vi "purge_v01.vi"(2 "Debug Mode":bool, 3 "Elapsed Time(s)":dbl, 4 "State":enum16{"Edit", "Start", "Run", "End", "Idle"}(ring), 5 "Argument List In":string[](array[string])) -> (0 "Status Out":string, 1 "Argument List Out":string[](array[string]))   [LabVIEW 2011]
panel:
  out "first":bool=TRUE
  out "total time":dbl
  out "is OK?":bool
  out "AsH3?":bool
  out "PH3?":bool
  out "In?":bool
  out "Ga?":bool
  out "Al?":bool
  in  "AsH3 Flow":dbl caption="AsH3 Flow (0-10 sccm)" format="%.2f"
  in  "P Flow":dbl caption="P Flow (0-100 sccm)" format="%.2f"
  in  "In Flow":dbl caption="In Flow (0-100 sscm)" format="%.2f"
  in  "Ga Flow":dbl caption="Ga Flow (0-10 sscm)" format="%.2f"
  in  "Al Flow":dbl caption="Al Flow (0-100 sscm)" format="%.2f"
  in  "Cancel":bool
  in  "OK":bool
  out "tTotal(s) 2":dbl
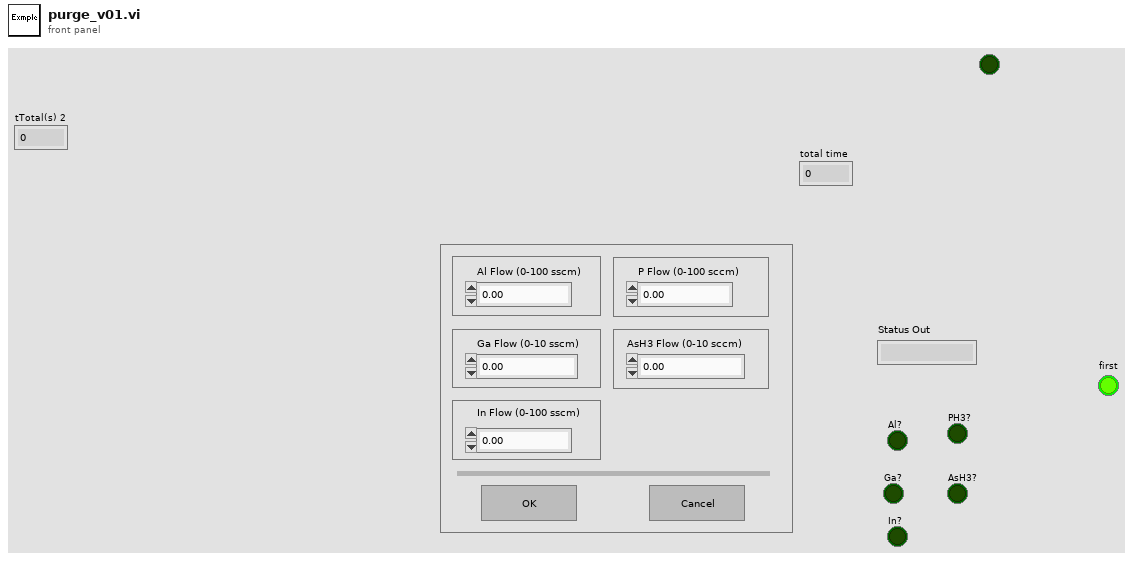
[diagram p1: front panel]
types:
  T1 = enum16{"Discrete", "Continuous", "Instantaneous", "Finite"}
  T2 = enum32{"Invalid", "Default", "Floating", "Floating/Auto-Hide", "Modal"}
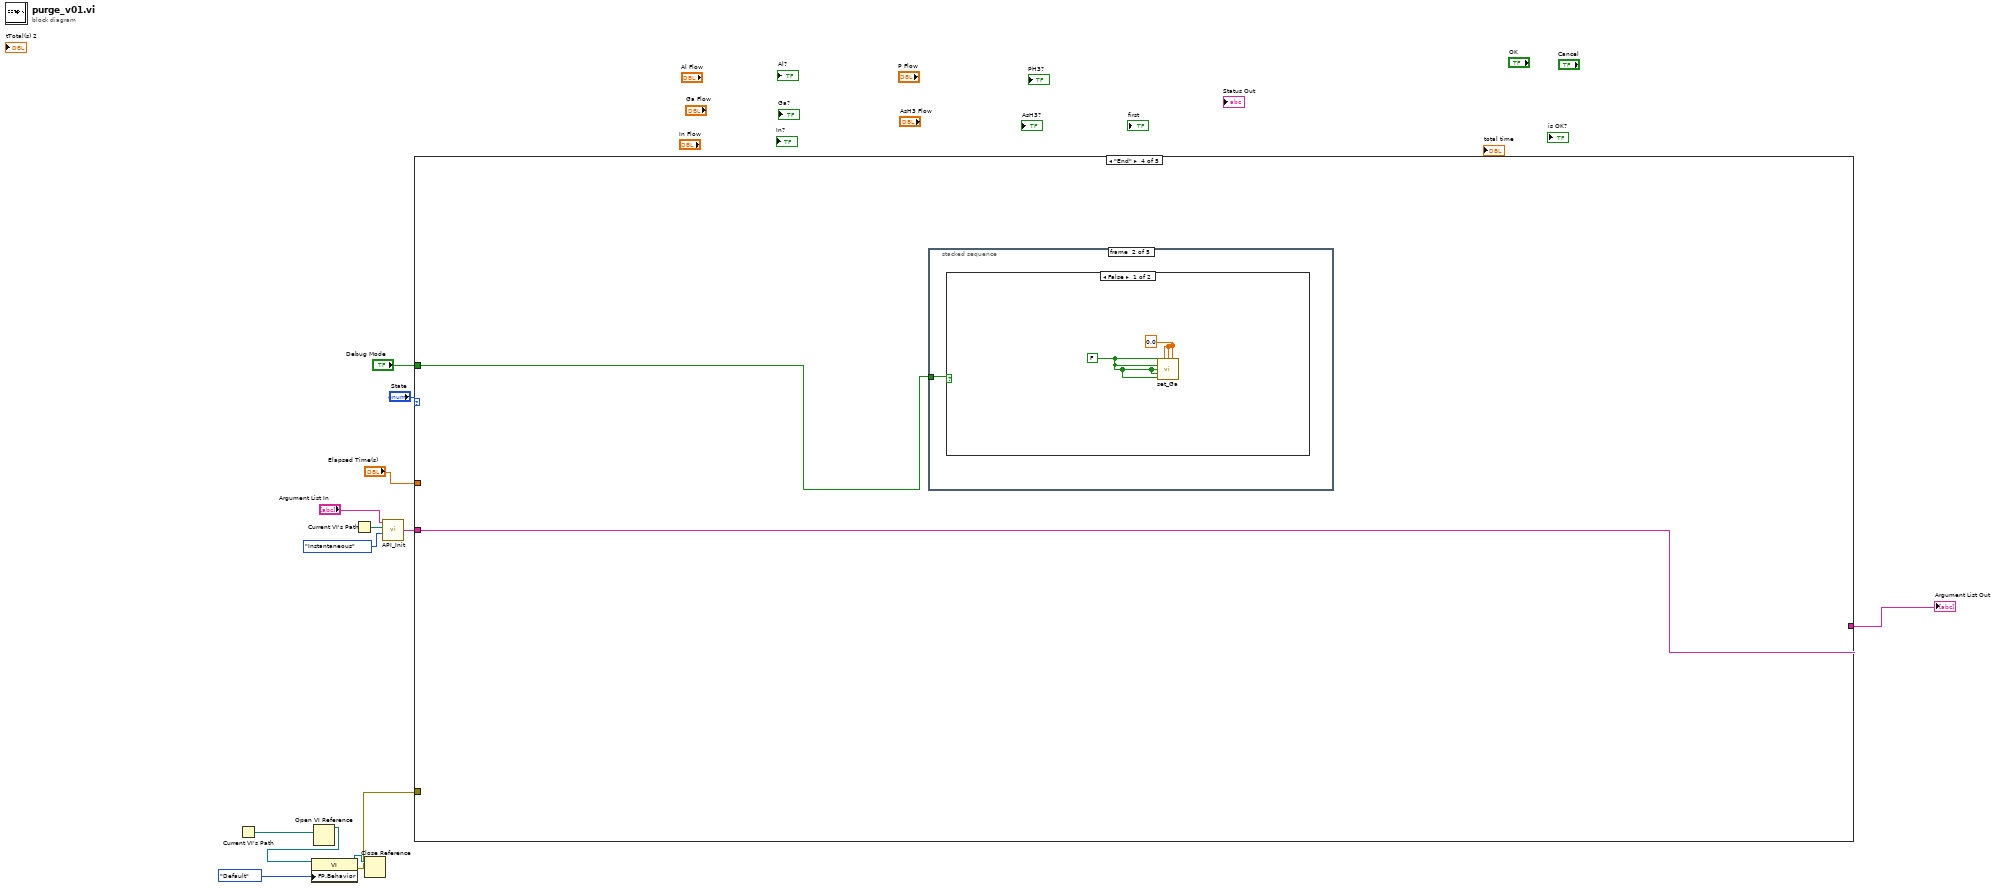
[diagram p0: block diagram]
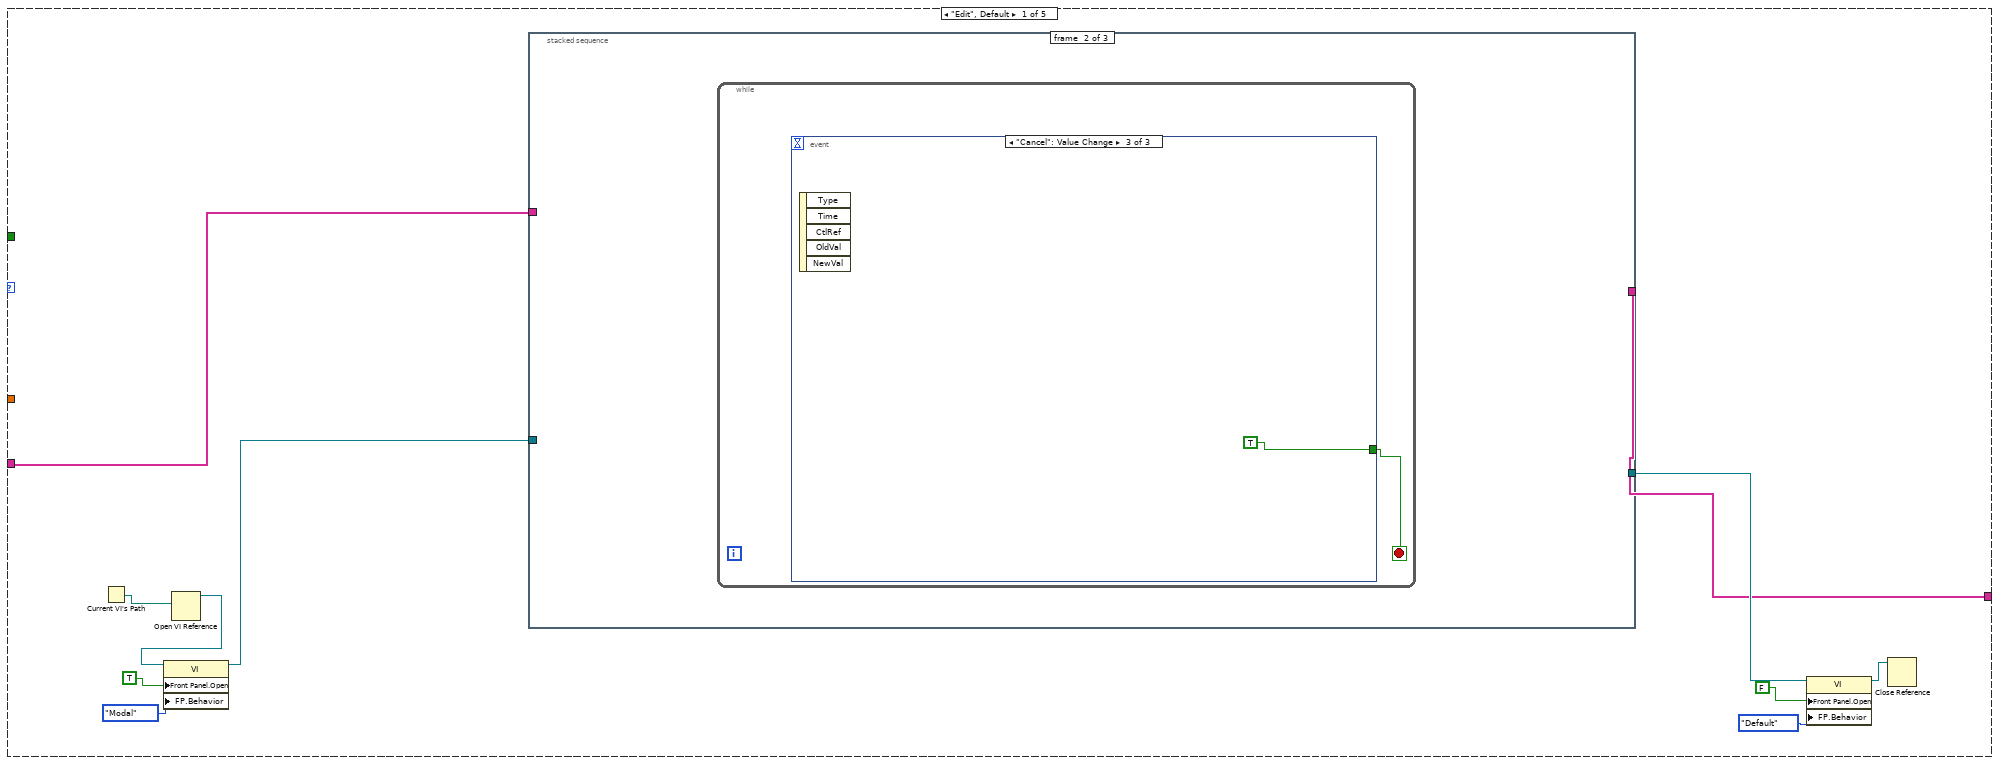
[diagram p2: hidden frame]
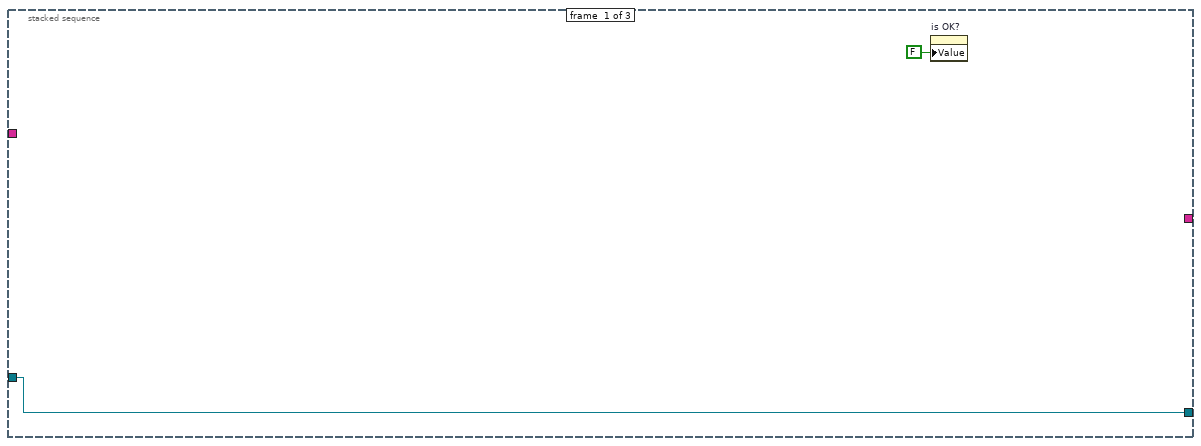
[diagram p3: hidden frame]
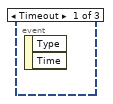
[diagram p4: hidden frame]
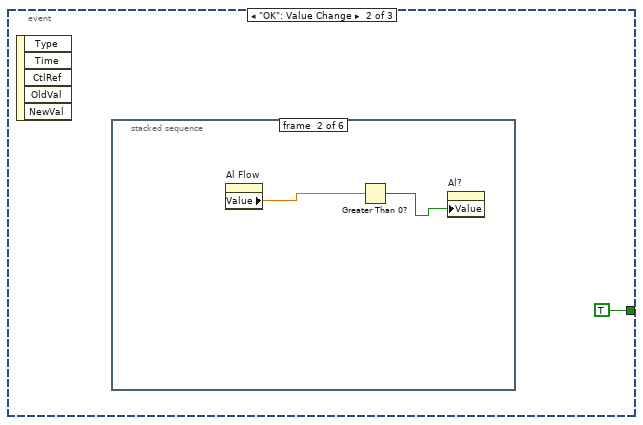
[diagram p5: hidden frame]
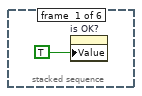
[diagram p6: hidden frame]
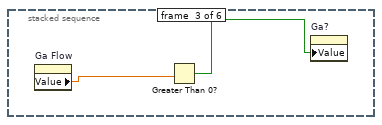
[diagram p7: hidden frame]
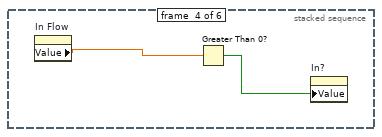
[diagram p8: hidden frame]
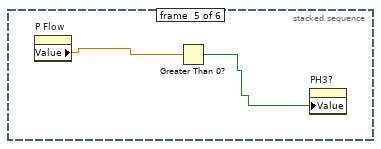
[diagram p9: hidden frame]
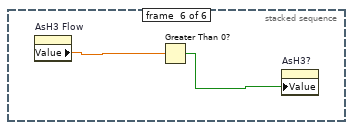
[diagram p10: hidden frame]
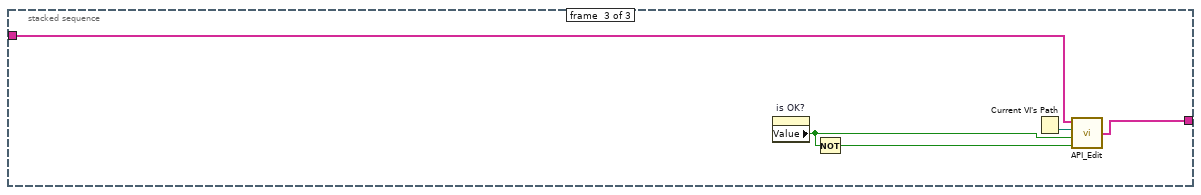
[diagram p11: hidden frame]
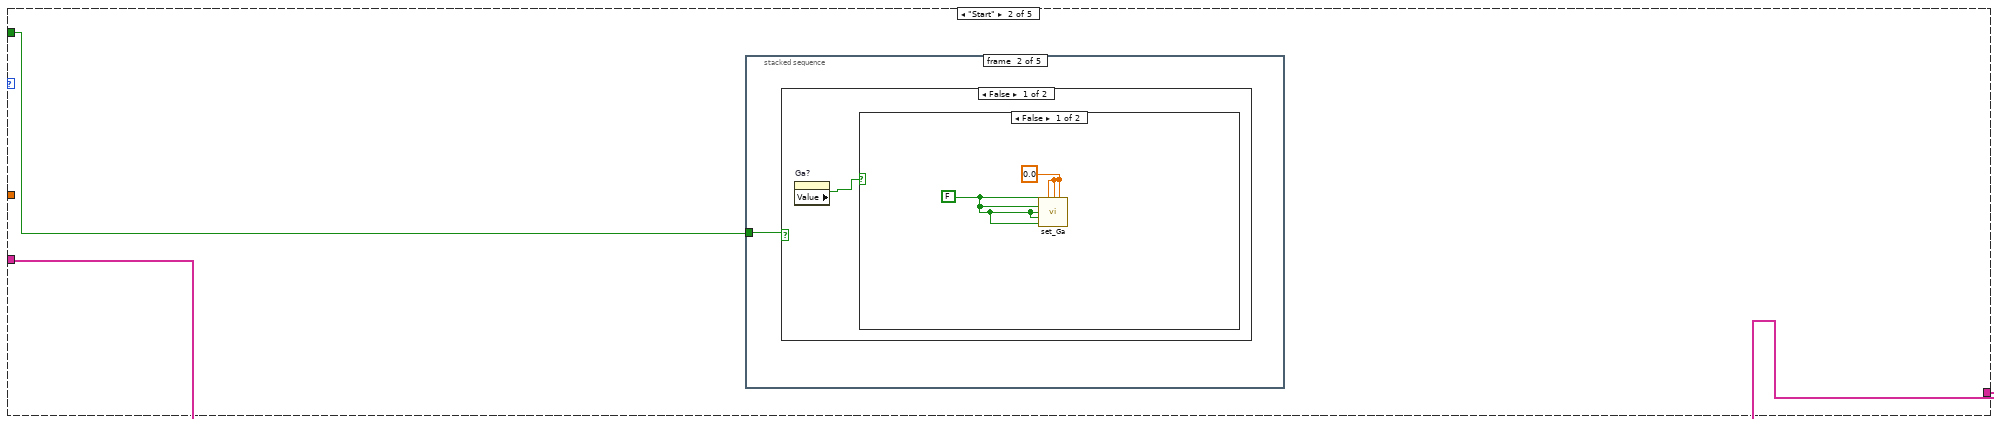
[diagram p12: hidden frame]
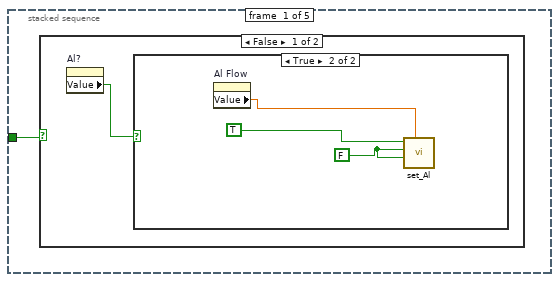
[diagram p13: hidden frame]
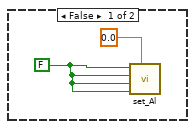
[diagram p14: hidden frame]
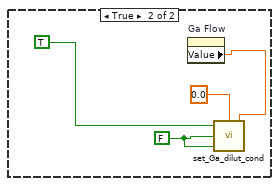
[diagram p16: hidden frame]
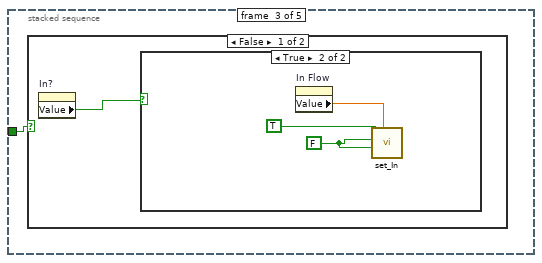
[diagram p18: hidden frame]
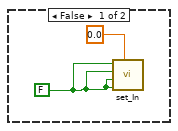
[diagram p19: hidden frame]
diagram:
  n1 = Current VI's Path() -> (path=w9:path)
  n2 = Open VI Reference(vi path=w9) -> (vi reference=w8:refnum<vi>)  [unwired: 1 in, 5 out]
  n3 = property class="VI"(reference=w8, "FP.Behavior"=T2."Default" ("Front Panel Window:Behavior")) -> (reference out=w6:refnum<vi>, error out=w5:errorcluster)  [unwired: 1 in]
  n4 = Current VI's Path() -> (path=w4:path)
  n5 = Close Reference(reference=w6) -> ()  [unwired: 1 in, 1 out]
  n6 = call "API_Init.vi"("API Mode"=T1."Instantaneous", "VI Path"=w4, "Argument List In"="Argument List In") -> ("Argument List Out"=w1:string[])  [unwired: 1 in]
  n7 = case shown="\"End\"" "State" {
    tunnel: "Debug Mode" -> [_ w47 _ w85 _]
    tunnel: "Elapsed Time(s)" -> [_ _ _ _ _]
    tunnel: w1 -> [w15 w46 w84 w86 w102]
    tunnel: [w14 w46 w84 w86 w102] -> w10
    tunnel: w5 -> [_ _ _ _ _]
    frame "Edit", Default {
      n8 = Current VI's Path() -> (path=w20:path)
      n9 = Open VI Reference(vi path=w20) -> (vi reference=w19:refnum<vi>)  [unwired: 1 in, 5 out]
      n10 = property class="VI"(reference=w19, "Front Panel.Open"=TRUE ("Front Panel Window:Open"), "FP.Behavior"=T2."Modal" ("Front Panel Window:Behavior")) -> (reference out=w18:refnum<vi>)  [unwired: 1 in, 1 out]
      n11 = stacked-sequence {
        tunnel: w15 -> [_ _ w41]
        tunnel: w18 -> [w26 _ _]
        tunnel: [w26 _ _] -> w22
        tunnel: [_ _ w43] -> w14
        frame #0 {
          n12 = property on="is OK?" class="Bool (strict)"("Value"=FALSE ("is OK?")) -> ()  [unwired: 2 in, 2 out]
        }
        frame #1 {
          n13 = while {
            stop <- w27 stop-if-true
            n14 = event shown="[2] \"Cancel\": Value Change" {
              selector: _ -> [_ _ _]
              dyn-events: _ -> [_ _ _]
              timeout: _ -> [_ _ _]
              tunnel: [_ TRUE TRUE] -> w27
              event Timeout {
                n15 = event-data() -> ()  [unwired: 1 in, 2 out]
              }
              event "OK": Value Change {
                n16 = event-data() -> ()  [unwired: 1 in, 5 out]
                n17 = stacked-sequence {
                  frame #0 {
                    n18 = property on="is OK?" class="Bool (strict)"("Value"=TRUE ("is OK?")) -> ()  [unwired: 2 in, 2 out]
                  }
                  frame #1 {
                    n19 = property on="Al Flow" class="DigNum (strict)"() -> ("Value"=w31:dbl)  [unwired: 2 in, 2 out]
                    n20 = Greater Than 0?(x=w31) -> (x > 0?=w30:bool)
                    n21 = property on="Al?" class="Bool (strict)"("Value"=w30) -> ()  [unwired: 2 in, 2 out]
                  }
                  frame #2 {
                    n22 = property on="Ga Flow" class="DigNum (strict)"() -> ("Value"=w33:dbl)  [unwired: 2 in, 2 out]
                    n23 = Greater Than 0?(x=w33) -> (x > 0?=w32:bool)
                    n24 = property on="Ga?" class="Bool (strict)"("Value"=w32) -> ()  [unwired: 2 in, 2 out]
                  }
                  frame #3 {
                    n25 = property on="In Flow" class="DigNum (strict)"() -> ("Value"=w35:dbl)  [unwired: 2 in, 2 out]
                    n26 = Greater Than 0?(x=w35) -> (x > 0?=w34:bool)
                    n27 = property on="In?" class="Bool (strict)"("Value"=w34) -> ()  [unwired: 2 in, 2 out]
                  }
                  frame #4 {
                    n28 = property on="P Flow" class="DigNum (strict)"() -> ("Value"=w37:dbl)  [unwired: 2 in, 2 out]
                    n29 = Greater Than 0?(x=w37) -> (x > 0?=w36:bool)
                    n30 = property on="PH3?" class="Bool (strict)"("Value"=w36) -> ()  [unwired: 2 in, 2 out]
                  }
                  frame #5 {
                    n31 = property on="AsH3 Flow" class="DigNum (strict)"() -> ("Value"=w39:dbl)  [unwired: 2 in, 2 out]
                    n32 = Greater Than 0?(x=w39) -> (x > 0?=w38:bool)
                    n33 = property on="AsH3?" class="Bool (strict)"("Value"=w38) -> ()  [unwired: 2 in, 2 out]
                  }
                }
              }
              event "Cancel": Value Change {
                n34 = event-data() -> ()  [unwired: 1 in, 5 out]
              }
            }
          }
        }
        frame #2 {
          n35 = property on="is OK?" class="Bool (strict)"() -> ("Value"=w42:bool)  [unwired: 2 in, 2 out]
          n36 = Not(x=w42) -> (.not. x?=w45:bool)
          n37 = Current VI's Path() -> (path=w44:path)
          n38 = call "API_Edit.vi"("Cancel"=w45, "OK"=w42, "VI Path"=w44, "Argument List In"=w41) -> ("Argument List Out"=w43:string[])
        }
      }
      n39 = property class="VI"(reference=w22, "Front Panel.Open"=FALSE ("Front Panel Window:Open"), "FP.Behavior"=T2."Default" ("Front Panel Window:Behavior")) -> (reference out=w23:refnum<vi>)  [unwired: 1 in, 1 out]
      n40 = Close Reference(reference=w23) -> ()  [unwired: 1 in, 1 out]
    }
    frame "Start" {
      n41 = stacked-sequence {
        tunnel: w47 -> [w48 w55 w63 w70 w77]
        frame #0 {
          n42 = case shown="False" w48 {
            frame False {
              n43 = property on="Al?" class="Bool (strict)"() -> ("Value"=w49:bool)  [unwired: 2 in, 2 out]
              n44 = case shown="True" w49 {
                frame False {
                  w50 = FALSE ("Al Active")
                  n45 = call "set_Al.vi"("Aluminum Flow"=0.0, "Al Remote"=w50, "Al Run"=w50, "Al Bubbler"=w50, "Al Active"=w50) -> ()  [unwired: 5 out]
                }
                frame True {
                  w52 = FALSE ("Al Bubbler")
                  n46 = property on="Al Flow" class="DigNum (strict)"() -> ("Value"=w53:dbl)  [unwired: 2 in, 2 out]
                  n47 = call "set_Al.vi"("Aluminum Flow"=w53, "Al Run"=w52, "Al Bubbler"=w52, "Al Active"=TRUE) -> ()  [unwired: 1 in, 5 out]
                }
              }
            }
            frame True {
            }
          }
        }
        frame #1 {
          n48 = case shown="False" w55 {
            frame False {
              n49 = property on="Ga?" class="Bool (strict)"() -> ("Value"=w56:bool)  [unwired: 2 in, 2 out]
              n50 = case shown="False" w56 {
                frame False {
                  w58 = FALSE ("Ga Active")
                  w57 = 0.0 ("Ga Flow 1")
                  n51 = call "set_Ga.vi"("Ga Active"=w58, "Ga Flow 3"=w57, "Ga Flow 2"=w57, "Ga Flow 1"=w57, "Ga Bubbler"=w58, "Ga H2 Dilute"=w58, "Ga Run"=w58, "Ga Remote"=w58) -> ()  [unwired: 8 out]
                }
                frame True {
                  w59 = FALSE ("Bubbler In")
                  n52 = property on="Ga Flow" class="DigNum (strict)"() -> ("Value"=w60:dbl)  [unwired: 2 in, 2 out]
                  n53 = call "set_Ga_dilut_cond.vi"("Ga flow (0-10 sccm)"=w60, "fDilution"=0.0, "Run"=w59, "Bubbler In"=w59, "Active"=TRUE ("Ga Active")) -> ()
                }
              }
            }
            frame True {
            }
          }
        }
        frame #2 {
          n54 = case shown="False" w63 {
            frame False {
              n55 = property on="In?" class="Bool (strict)"() -> ("Value"=w64:bool)  [unwired: 2 in, 2 out]
              n56 = case shown="True" w64 {
                frame False {
                  w66 = FALSE ("In Remote")
                  n57 = call "set_In.vi"("Indium Flow"=0.0, "In Remote"=w66, "In Run"=w66, "In Bubbler"=w66, "In Active"=w66) -> ()  [unwired: 5 out]
                }
                frame True {
                  w67 = FALSE ("In Bubbler")
                  n58 = property on="In Flow" class="DigNum (strict)"() -> ("Value"=w68:dbl)  [unwired: 2 in, 2 out]
                  n59 = call "set_In.vi"("Indium Flow"=w68, "In Run"=w67, "In Bubbler"=w67, "In Active"=TRUE ("In Run")) -> ()  [unwired: 1 in, 5 out]
                }
              }
            }
            frame True {
            }
          }
        }
        frame #3 {
          n60 = case shown="False" w70 {
            frame False {
              n61 = property on="PH3?" class="Bool (strict)"() -> ("Value"=w71:bool)  [unwired: 2 in, 2 out]
              n62 = case shown="True" w71 {
                frame False {
                  w72 = FALSE ("P_Gas Active")
                  n63 = call "set_P_gas.vi"("P_Gas Active"=w72, "P_Gas Flow"=0.0, "P_Gas In"=w72, "P_Gas H2 In"=w72, "P_Gas Run"=w72, "P_Gas Remote"=w72) -> ()  [unwired: 10 out]
                }
                frame True {
                  w74 = FALSE ("P_Gas In")
                  w75 = TRUE ("P_Gas Active")
                  n64 = property on="P Flow" class="DigNum (strict)"() -> ("Value"=w76:dbl)  [unwired: 2 in, 2 out]
                  n65 = call "set_P_gas.vi"("P_Gas Active"=w75, "P_Gas Flow"=w76, "P_Gas In"=w74, "P_Gas H2 In"=w75, "P_Gas Run"=w74) -> ()  [unwired: 1 in, 10 out]
                }
              }
            }
            frame True {
            }
          }
        }
        frame #4 {
          n66 = case shown="False" w77 {
            frame False {
              n67 = property on="AsH3?" class="Bool (strict)"() -> ("Value"=w78:bool)  [unwired: 2 in, 2 out]
              n68 = case shown="True" w78 {
                frame False {
                  w79 = FALSE ("As_Gas Active")
                  n69 = call "set_As_gas.vi"("As_Gas Active"=w79, "As_Gas Flow"=0.0, "As_Gas In"=w79, "As_Gas H2"=w79, "As_Gas Run"=w79, "As_Gas Remote"=w79) -> ()  [unwired: 10 in]
                }
                frame True {
                  w81 = FALSE ("As_Gas In")
                  w82 = TRUE ("As_Gas Active")
                  n70 = property on="AsH3 Flow" class="DigNum (strict)"() -> ("Value"=w83:dbl)  [unwired: 2 in, 2 out]
                  n71 = call "set_As_gas.vi"("As_Gas Active"=w82, "As_Gas Flow"=w83, "As_Gas In"=w81, "As_Gas H2"=w82, "As_Gas Run"=w81) -> ()  [unwired: 11 in]
                }
              }
            }
            frame True {
            }
          }
        }
      }
    }
    frame "Run" {
    }
    frame "End" {
      n72 = stacked-sequence {
        tunnel: w85 -> [w87 w90 w93 w96 w99]
        frame #0 {
          n73 = case shown="False" w87 {
            frame False {
              w89 = FALSE ("Al Active")
              n74 = call "set_Al.vi"("Aluminum Flow"=0.0, "Al Remote"=w89, "Al Run"=w89, "Al Bubbler"=w89, "Al Active"=w89) -> ()  [unwired: 5 out]
            }
            frame True {
            }
          }
        }
        frame #1 {
          n75 = case shown="False" w90 {
            frame False {
              w92 = FALSE ("Ga Active")
              w91 = 0.0 ("Ga Flow 1")
              n76 = call "set_Ga.vi"("Ga Active"=w92, "Ga Flow 3"=w91, "Ga Flow 2"=w91, "Ga Flow 1"=w91, "Ga Bubbler"=w92, "Ga H2 Dilute"=w92, "Ga Run"=w92, "Ga Remote"=w92) -> ()  [unwired: 8 out]
            }
            frame True {
            }
          }
        }
        frame #2 {
          n77 = case shown="False" w93 {
            frame False {
              w95 = FALSE ("In Remote")
              n78 = call "set_In.vi"("Indium Flow"=0.0, "In Remote"=w95, "In Run"=w95, "In Bubbler"=w95, "In Active"=w95) -> ()  [unwired: 5 out]
            }
            frame True {
            }
          }
        }
        frame #3 {
          n79 = case shown="False" w96 {
            frame False {
              w97 = FALSE ("P_Gas Active")
              n80 = call "set_P_gas.vi"("P_Gas Active"=w97, "P_Gas Flow"=0.0, "P_Gas In"=w97, "P_Gas H2 In"=w97, "P_Gas Run"=w97, "P_Gas Remote"=w97) -> ()  [unwired: 10 out]
            }
            frame True {
            }
          }
        }
        frame #4 {
          n81 = case shown="False" w99 {
            frame False {
              w100 = FALSE ("As_Gas Active")
              n82 = call "set_As_gas.vi"("As_Gas Active"=w100, "As_Gas Flow"=0.0, "As_Gas In"=w100, "As_Gas H2"=w100, "As_Gas Run"=w100, "As_Gas Remote"=w100) -> ()  [unwired: 10 in]
            }
            frame True {
            }
          }
        }
      }
    }
    frame "Idle" {
    }
  }
  "Argument List Out" <- w10
